vi "SetBit(U64).vi"(8 "error in (no error)":errorcluster caption="错误输入（无错误）", 10 "Bit(0-63)":u8, 11 "Input(U64)":u64 format="%.0x") -> (0 "error out":errorcluster caption="错误输出", 3 "Output(64)":u64 format="%.0x")   [LabVIEW 2012]
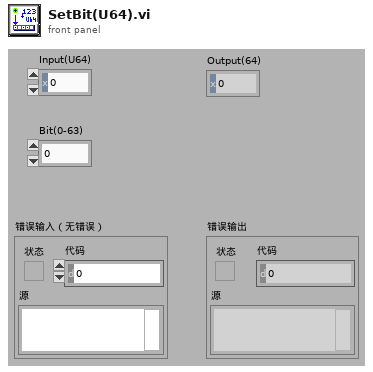
[diagram p1: front panel]
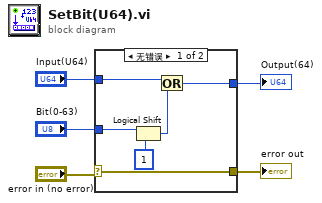
[diagram p0: block diagram]
diagram:
  n1 = case shown="无错误" "error in (no error)" {
    selector: "error in (no error)" -> [w11 w12]
    tunnel: [w11 w12] -> w4
    tunnel: "Bit(0-63)" -> [w9 _]
    tunnel: "Input(U64)" -> [w8 _]
    tunnel: [w6 _] -> w1
    frame No Error {
      n2 = Logical Shift(y=w9, x=u64 1) -> (x << y=w7:u64)
      n3 = Or(x=w8, y=w7) -> (x .or. y?=w6:u64)
    }
    frame Error {
    }
  }
  "error out" <- w4
  "Output(64)" <- w1
